vi "alg.vi"(1 "24-bit pixmap":u32[][](array[numeric])) -> (0 "Array 2":i32[][](array[numeric]))   [LabVIEW 2016]
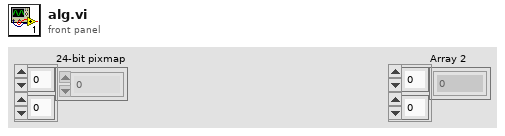
[diagram p1: front panel]
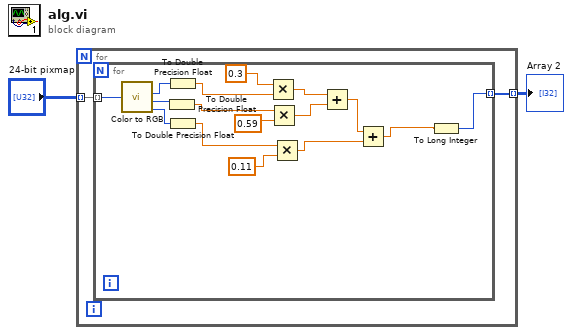
[diagram p0: block diagram]
diagram:
  n1 = for {
    tunnel: "24-bit pixmap" -> [w4] mode=indexing
    tunnel: [w3] -> w2 mode=indexing
    n2 = for {
      tunnel: w4 -> [w20] mode=indexing
      tunnel: [w5] -> w3 mode=indexing
      n3 = call <vilib>:"Color to RGB.vi"("Color"=w20) -> ("R"=w12:u8, "G"=w10:u8, "B"=w8:u8)  [unwired: 1 out]
      n4 = To Double Precision Float(number=w10) -> (double precision float=w9:dbl)
      n5 = To Double Precision Float(number=w12) -> (double precision float=w11:dbl)
      n6 = To Double Precision Float(number=w8) -> (double precision float=w7:dbl)
      n7 = Multiply(x=0.3, y=w11) -> (x*y=w16:dbl)
      n8 = Multiply(x=w9, y=0.59) -> (x*y=w15:dbl)
      n9 = Multiply(x=w7, y=0.11) -> (x*y=w14:dbl)
      n10 = Add(x=w16, y=w15) -> (x+y=w13:dbl)
      n11 = Add(x=w13, y=w14) -> (x+y=w6:dbl)
      n12 = To Long Integer(number=w6) -> (32bit integer=w5:i32)
    }
  }
  "Array 2" <- w2
